vi "Excel Get Last Row.vi"(0 "report in":refnum<class "NI_report.lvclass">, 7 "offset":i32, 11 "error in (no error)":errorcluster, 12 "MS Office parameters":T1) -> (4 "report out":refnum<class "NI_report.lvclass">, 14 "MS Office parameters out":T1, 15 "error out":errorcluster)   [LabVIEW 2010, in "NI_Excel.lvclass"]
doc: "Retrieves the coordinates of the last row in an Excel worksheet. Use the <B>MS Office parameters</B> input to append the contents of the row to a report."
uses:
  <vilib>/Utility/NIReport.llb/Excel/NI_Excel.lvclass
  <vilib>/Utility/NIReport.llb/NI_report.lvclass
  <vilib>/Utility/NIReport.llb/Excel/NI_Excel.lvclass/NI_Excel.ctl
  <vilib>/addons/_office/NI_ReportGenerationToolkit.lvlib
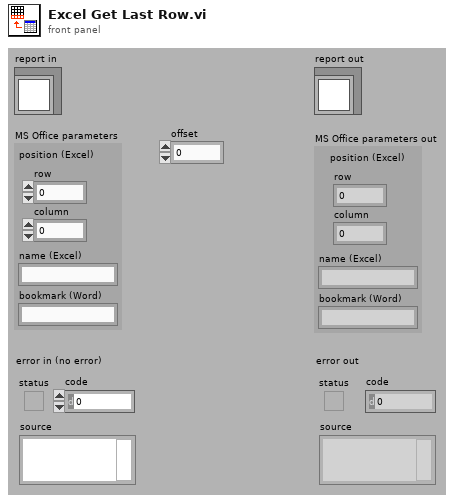
[diagram p1: front panel]
types:
  T1 = cluster{"position (Excel)":cluster{"row":i32, "column":i32}, "name (Excel)":string, "bookmark (Word)":string}
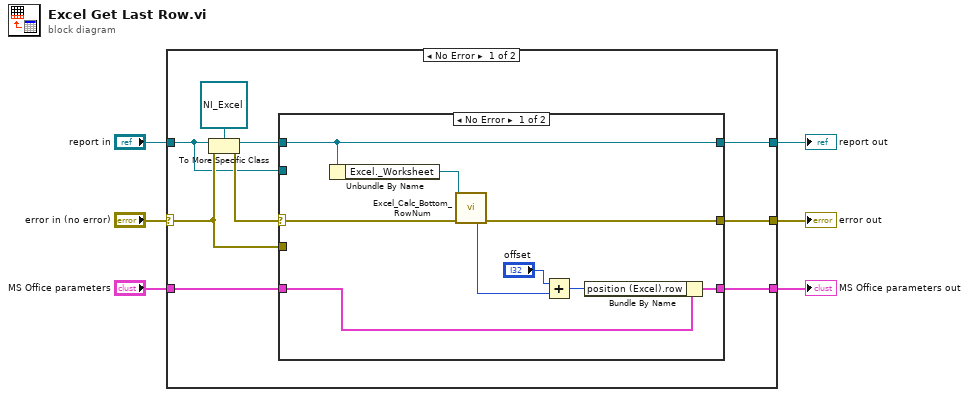
[diagram p0: block diagram]
diagram:
  n1 = case shown="No Error" "error in (no error)" {
    selector: "error in (no error)" -> [w10 w29]
    tunnel: "report in" -> [w7 w30]
    tunnel: [w8 w30] -> w5
    tunnel: [w13 w29] -> w4
    tunnel: "MS Office parameters" -> [w15 w28]
    tunnel: [w14 w28] -> w2
    frame No Error {
      n2 = To More Specific Class(target class=refnum<class "NI_Excel.lvclass"> refnum ("report in"), reference=w7, error in=w10) -> (specific class reference=w9:refnum<class "NI_Excel.lvclass">, error out=w11:errorcluster)
      n3 = case shown="No Error" w11 {
        selector: w11 -> [w17 _]
        tunnel: w15 -> [w24 w27]
        tunnel: [w23 w27] -> w14
        tunnel: [w18 w26] -> w13
        tunnel: w9 -> [w16 _]
        tunnel: w10 -> [_ w26]
        tunnel: [w16 w25] -> w8
        tunnel: w7 -> [_ w25]
        frame No Error {
          n4 = Unbundle By Name(w16) -> ("Excel._Worksheet"=w19:refnum<k7>)
          n5 = call <vilib>:"Excel_Calc_Bottom_RowNum.vi"("Excel._Worksheet In"=w19, "error in (no error)"=w17) -> ("bottom row#"=w20:i32, "error out"=w18:errorcluster)  [unwired: 12 out]
          n6 = Add(x="offset", y=w20) -> (x+y=w21:i32)
          n7 = Bundle By Name(cluster=w24, "position (Excel).row"=w21) -> (w23:T1)
        }
        frame Error {
        }
      }
    }
    frame Error {
    }
  }
  "error out" <- w4
  "report out" <- w5
  "MS Office parameters out" <- w2
